vi "Self Event Alias.vi"(11 "Event jettl in":refnum<class "Event jettl.lvclass">) -> (2 "Self Event Alias":string)   [LabVIEW 2021, in "jettl.lvlib" / "Event jettl.lvclass"]
uses:
  Event jettl.lvclass
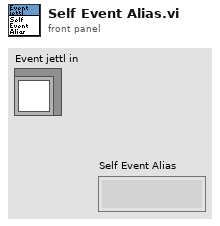
[diagram p1: front panel]
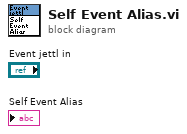
[diagram p0: block diagram]
diagram:
